vi "Survey.vi"() -> ()   [LabVIEW 2016]
panel:
  out "concatenated string":string
  in  "Tab Control":T1(tab)
  out "Images can be found in this folder:":string
  in  "?":bool
  in  "?":bool
  in  "Module Number":dbl
  in  "Stave Name":string
  out "Error":string
  out "Survey Results (Tables)":string
  out "Delta X Histogram":picture
  out "Delta Y Histogram":picture
  out "Angle Over Time":picture
  out "Relative Position Over Time":picture
  # "Select all functions you would like to execute"
  # "-> Copy the survey files from original folders to compiled folder"
  # "General Folder of the Stave where you can find all the Calibrations Directories"
  # "-> Generate and display results and graphs"
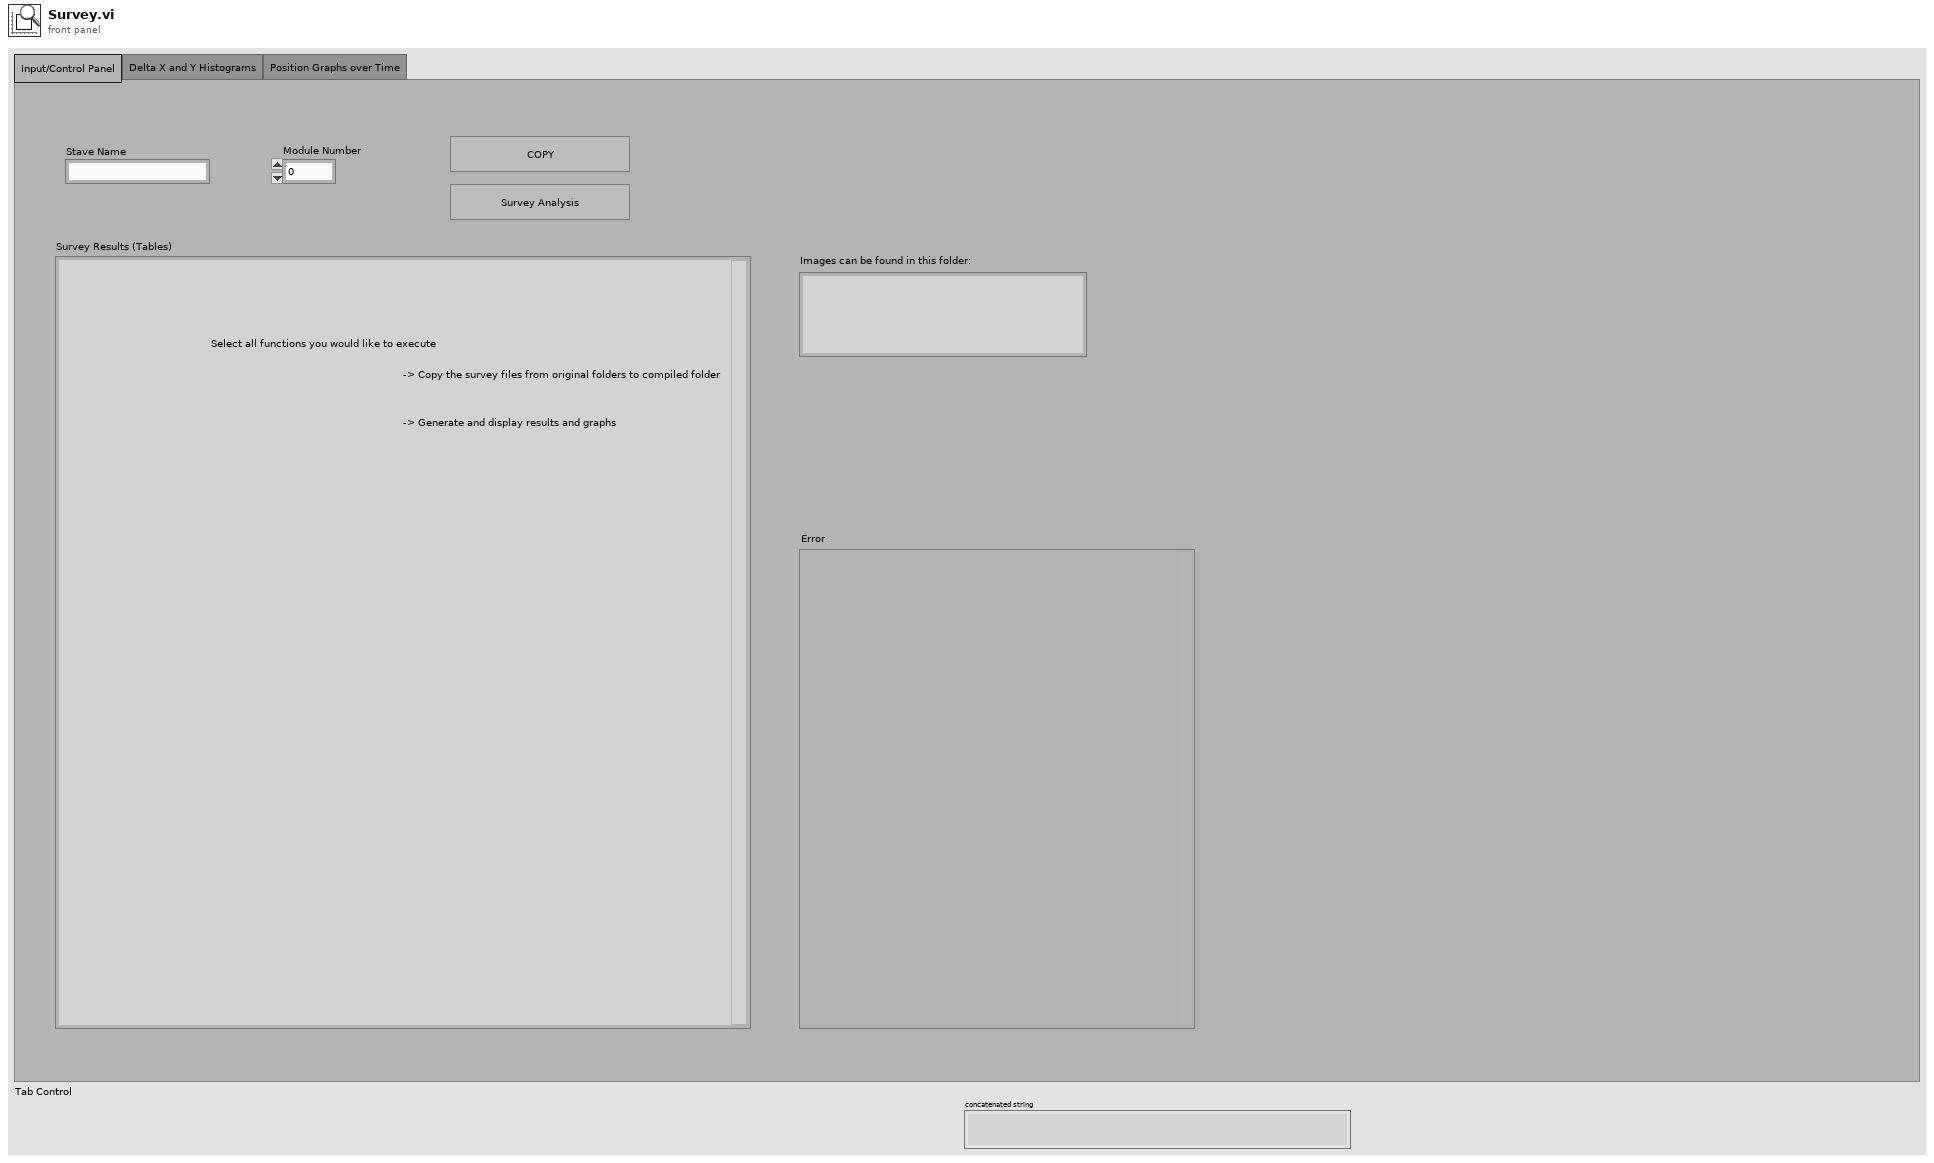
[diagram p1: front panel]
types:
  T1 = enum32{"Input/Control Panel", "Delta X and Y Histograms", "Position Graphs over Time"}
  T2 = typedef "imagedata.ctl" = cluster{"image type":i32, "image depth":i32, "image":u8[], "mask":u8[], "colors":u32[], "Rectangle":cluster{"left":i16, "top":i16, "right":i16, "bottom":i16}}
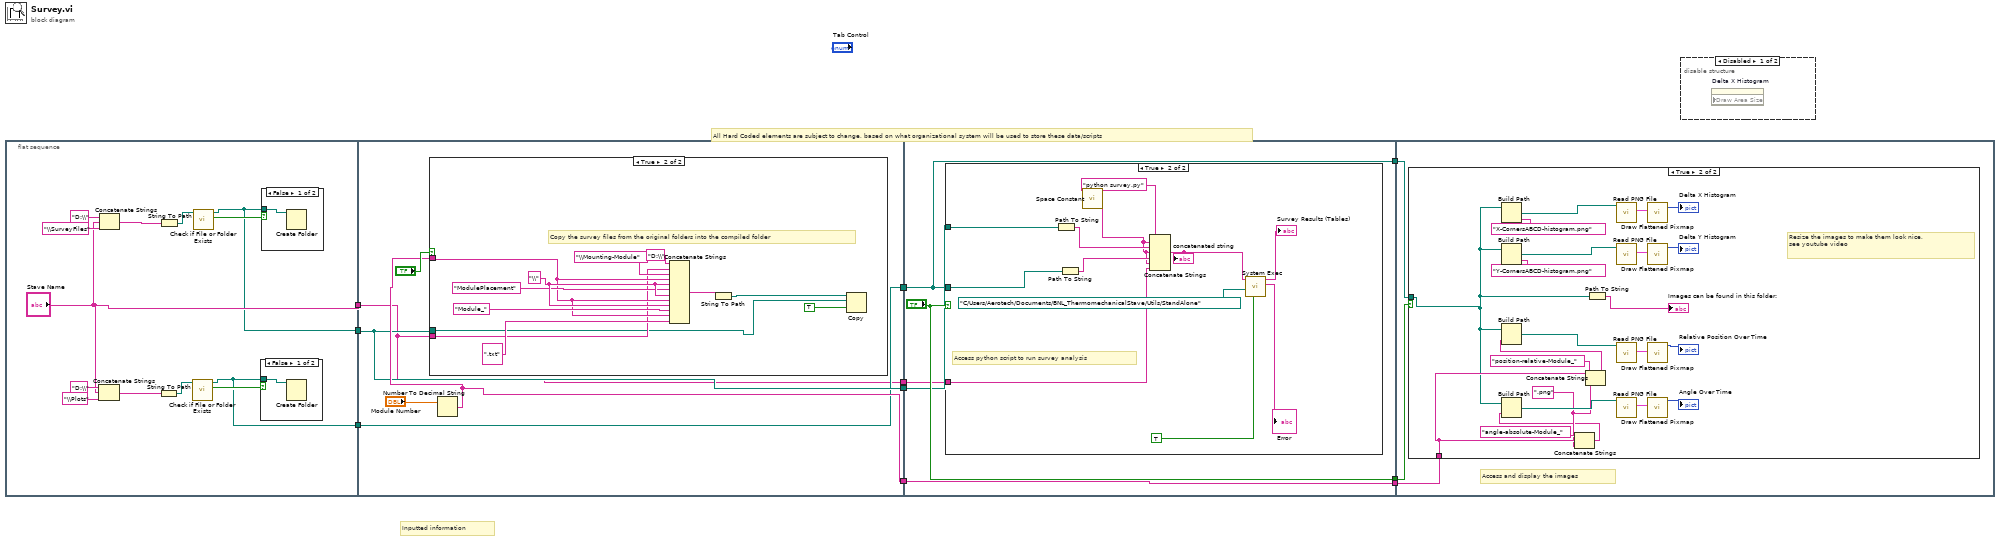
[diagram p0: block diagram]
diagram:
  # "Inputted information"
  # "All Hard Coded elements are subject to change, based on what organizational system will be used to store these data/scripts"
  n1 = flat-sequence {
    tunnel: ["Stave Name"] -> w7
    tunnel: [w12] -> w6
    tunnel: [w11] -> w3
    tunnel: [w29] -> w9
    tunnel: w7 -> [w26]
    tunnel: w6 -> [w28]
    tunnel: [w28] -> w5
    tunnel: [w27] -> w4
    tunnel: w3 -> [w27]
    tunnel: [w26] -> w1
    tunnel: ["?"] -> w10
    tunnel: w9 -> [w47]
    tunnel: [w47] -> w8
    tunnel: w5 -> [w46]
    tunnel: w4 -> [w45]
    tunnel: [w45] -> w2
    tunnel: w1 -> [w44]
    tunnel: w10 -> [w63]
    tunnel: w8 -> [w62]
    tunnel: w2 -> [w61]
    frame #0 {
      n2 = Concatenate Strings("D:\\" ("string"), "Stave Name", "\\Plots" ("string")) -> (w18:string)
      n3 = Concatenate Strings("D:\\" ("string"), "Stave Name", "\\SurveyFiles" ("string")) -> (w23:string)
      n4 = String To Path(string=w18) -> (path=w15:path)
      n5 = String To Path(string=w23) -> (path=w20:path)
      n6 = call <vilib>:"Check if File or Folder Exists.vi"("path"=w15) -> ("file or folder exists?"=w14:bool, "dup path"=w11:path)  [unwired: 8 in, 1 out]
      n7 = call <vilib>:"Check if File or Folder Exists.vi"("path"=w20) -> ("file or folder exists?"=w19:bool, "dup path"=w12:path)  [unwired: 8 in, 1 out]
      n8 = case shown="False" w14 {
        tunnel: w11 -> [w24 _]
        frame False {
          n9 = Create Folder(path (use dialog)=w24) -> ()  [unwired: 2 in, 3 out]
        }
        frame True {
        }
      }
      n10 = case shown="False" w19 {
        tunnel: w12 -> [w25 _]
        frame False {
          n11 = Create Folder(path (use dialog)=w25) -> ()  [unwired: 2 in, 3 out]
        }
        frame True {
        }
      }
    }
    frame #1 {
      n12 = Number To Decimal String(number="Module Number") -> (decimal integer string=w29:string)  [unwired: 1 in]
      n13 = case shown="True" "?" {
        tunnel: w29 -> [_ w35]
        tunnel: w26 -> [_ w33]
        tunnel: w28 -> [_ w32]
        frame False {
        }
        frame True {
          w38 = "\\"
          # "Copy the survey files from the original folders into the compiled folder"
          n14 = Concatenate Strings("D:\\" ("string"), w33, "\\Mounting-Module" ("string"), w35, w38, "ModulePlacement", w38, w35, w38, "Module_", w35, ".txt") -> (w41:string)
          n15 = String To Path(string=w41) -> (path=w42:path)
          n16 = Copy(9:TRUE, 10:w32, 11:w42) -> ()  [unwired: 2 in, 3 out]
        }
      }
    }
    frame #2 {
      n17 = case shown="True" "?" {
        tunnel: w46 -> [_ w54]
        tunnel: w45 -> [_ w51]
        tunnel: w44 -> [_ w49]
        frame False {
        }
        frame True {
          # "Access python script to run survey analysis"
          n18 = Path To String(path=w54) -> (string=w57:string)
          n19 = Path To String(path=w51) -> (string=w52:string)
          n20 = call <vilib>:"Space Constant.vi"() -> ("String"=w50:string)
          n21 = Concatenate Strings("python survey.py" ("string"), w50, w57, w50, w52, w50, w49) -> (w60:string)
          "concatenated string" <- w60
          n22 = call <vilib>:"System Exec.vi"("run minimized? (F)"=TRUE, "working directory"=path "C:/Users/Aerotech/Documents/BNL_ThermomechanicalStave/Utils/StandAlone", "command line"=w60) -> ("standard error"=→"Error":string, "standard output"=→"Survey Results (Tables)":string)  [unwired: 5 in, 2 out]
        }
      }
    }
    frame #3 {
      # "Access and display the images"
      n23 = case shown="True" w63 {
        tunnel: w62 -> [_ w68]
        tunnel: w61 -> [_ w64]
        frame False {
        }
        frame True {
          w67 = ".png" ("string")
          # "Resize the images to make them look nice,\nsee youtube video"
          n24 = Build Path(base path=w64, name or relative path="X-CornersABCD-histogram.png") -> (appended path=w82:path)
          n25 = Build Path(base path=w64, name or relative path="Y-CornersABCD-histogram.png") -> (appended path=w78:path)
          n26 = Concatenate Strings("angle-absolute-Module_" ("name or relative path"), w68, w67) -> (w66:string)
          n27 = Build Path(base path=w64, name or relative path=w66) -> (appended path=w74:path)
          n28 = Concatenate Strings("position-relative-Module_", w68, w67) -> (w71:string)
          n29 = Build Path(base path=w64, name or relative path=w71) -> (appended path=w76:path)
          n30 = Path To String(path=w64) -> (string=→"Images can be found in this folder:":string)
          n31 = call <vilib>:"Read PNG File.vi"("path to PNG file"=w82) -> ("image data"=w85:T2)  [unwired: 8 in, 2 out]
          n32 = call <vilib>:"Read PNG File.vi"("path to PNG file"=w78) -> ("image data"=w80:T2)  [unwired: 8 in, 2 out]
          n33 = call <vilib>:"Read PNG File.vi"("path to PNG file"=w76) -> ("image data"=w77:T2)  [unwired: 8 in, 2 out]
          n34 = call <vilib>:"Read PNG File.vi"("path to PNG file"=w74) -> ("image data"=w75:T2)  [unwired: 8 in, 2 out]
          n35 = call <vilib>:"Draw Flattened Pixmap.vi"("image data"=w85) -> ("new picture"=→"Delta X Histogram":picture)  [unwired: 8 in]
          n36 = call <vilib>:"Draw Flattened Pixmap.vi"("image data"=w80) -> ("new picture"=→"Delta Y Histogram":picture)  [unwired: 8 in]
          n37 = call <vilib>:"Draw Flattened Pixmap.vi"("image data"=w77) -> ("new picture"=→"Relative Position Over Time":picture)  [unwired: 8 in]
          n38 = call <vilib>:"Draw Flattened Pixmap.vi"("image data"=w75) -> ("new picture"=→"Angle Over Time":picture)  [unwired: 8 in]
        }
      }
    }
  }
  n39 = disable-structure shown="Disabled" {
    frame Disabled {
      n40 = property on="Delta X Histogram" class="Pict" props=["Draw Area Size"]() -> ()  [unwired: 3 in, 2 out]
    }
    frame Enabled {
    }
  }
